vi "SVT Fractional Octave Filtering (N Ch).vi"(6 "reset filter (F)":bool, 7 "coerce to nearest standard midband frequency?":bool, 8 "error in (no error)":errorcluster, 9 "midband frequency":dbl, 10 "bandwidth":T1(ring), 11 "scaled signal(s)":waveform(dbl)[](array[waveform])) -> (0 "error out":errorcluster, 2 "actual midband frequency [Hz]":dbl, 3 "filtered signl(s)":waveform(dbl)[](array[waveform]), 4 "settled?":bool)   [LabVIEW 2017, in "SoundVib_Octave_2014 standard.lvlib"]
doc: "Performs fractional octave filtering on <B>scaled signal [EU]</B> in accordance with either the ANSI S1.11-2014 standard or the IEC 61260-1:2014 standard.\n\n \n\nYou can use this polymorphic VI to perform fractional octave filtering on a single channel or on N channels. The data type you wire to the <B>scaled signal [EU]</B> input determines the polymorphic instance to use."
uses:
  <vilib>/addons/Sound and Vibration/svt_Octave/SoundVib_Octave_2014 standard.lvlib
  <vilib>/addons/_NISVFA/_Shared subVIs/Controls/svc_Octave Standard.ctl
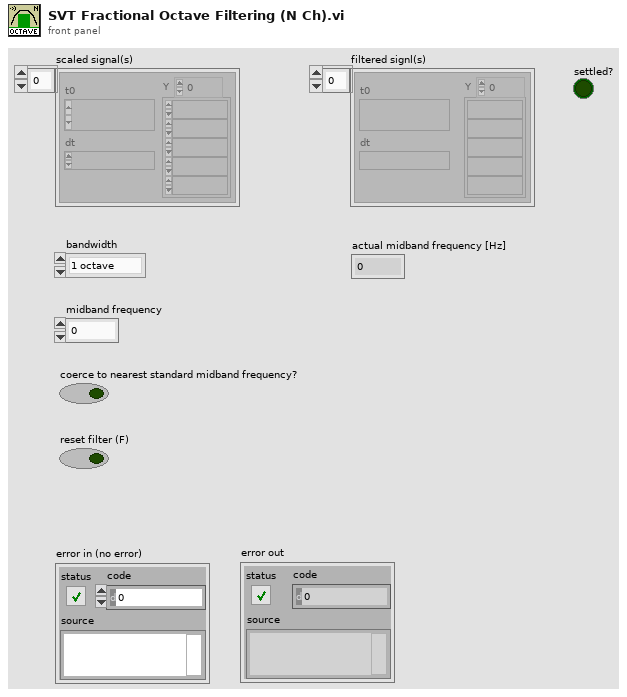
[diagram p1: front panel]
types:
  T1 = enum16{"1 octave", "1/3 octave", "1/6 octave", "1/12 octave", "1/24 octave"}
  T2 = typedef "svc_Octave Standard.ctl" = enum16{"ANSI S1.11", "IEC 61260"}
  T3 = cluster{"standard":T2, "bandwidth":enum16{"1 octave", "1/3 octave", "1/6 octave", "1/12 octave", "1/24 octave"}}
  T4 = cluster{"midband frequency":dbl, "coerce to nearest standard midband frequency?":bool}
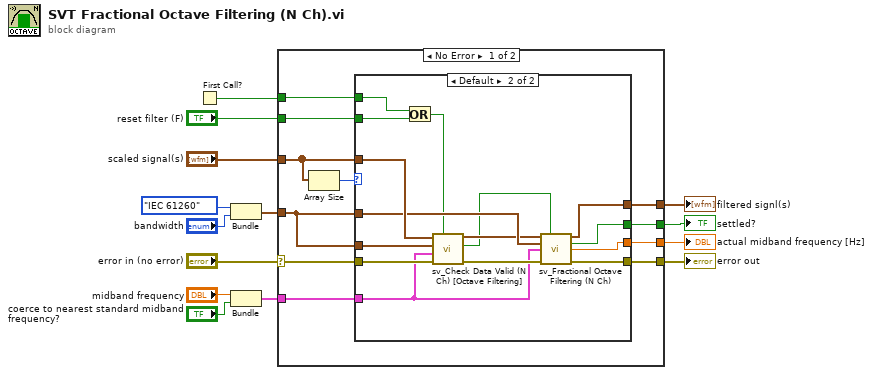
[diagram p0: block diagram]
diagram:
  n1 = First Call?() -> (First Call?: T/F=w11:bool)
  n2 = Bundle("standard"=svc_Octave_Standard."IEC 61260", "bandwidth"="bandwidth") -> (w5:T3)  [unwired: 1 in]
  n3 = Bundle("midband frequency"="midband frequency", "coerce to nearest standard midband frequency?"="coerce to nearest standard midband frequency?") -> (w2:T4)  [unwired: 1 in]
  n4 = case shown="No Error" "error in (no error)" {
    selector: "error in (no error)" -> [w25 w42]
    tunnel: [w16 w42] -> w13
    tunnel: "scaled signal(s)" -> [w24 _]
    tunnel: "reset filter (F)" -> [w22 _]
    tunnel: w5 -> [w20 _]
    tunnel: w2 -> [w19 _]
    tunnel: w11 -> [w21 _]
    tunnel: [w18 _] -> w8
    tunnel: [w17 _] -> w9
    tunnel: [w15 _] -> w1
    frame No Error {
      n5 = Array Size(array=w24) -> (size(s)=w23:i32)
      n6 = case shown="Default" w23 {
        tunnel: w25 -> [w26 w41]
        tunnel: w24 -> [_ w40]
        tunnel: w22 -> [_ w31]
        tunnel: w21 -> [_ w30]
        tunnel: w20 -> [_ w39]
        tunnel: w20 -> [_ w37]
        tunnel: w19 -> [_ w28]
        tunnel: [_ w34] -> w18
        tunnel: [_ w33] -> w17
        tunnel: [w26 w32] -> w16
        tunnel: [_ w27] -> w15
        frame 0 {
        }
        frame Default {
          n7 = Or(x=w30, y=w31) -> (x .or. y?=w29:bool)
          n8 = call <vilib>:"sv_Check Data Valid (N Ch) [Octave Filtering].vi"("reset filter (F)"=w29, "error in (no error)"=w41, "midband frequency setting"=w28, "1/n octave settings"=w39, "scaled signal(s)"=w40) -> ("error out"=w38:errorcluster, "reset filter"=w35:bool, "dup scaled signal(s)"=w36:waveform(dbl)[])  [unwired: 4 in]
          n9 = call <vilib>:"sv_Fractional Octave Filtering (N Ch).vi"("scaled signal(s) [EU]"=w36, "reset filter (F)"=w35, "1/n octave settings"=w37, "midband frequency setting"=w28, "error in (no error)"=w38) -> ("filtered signal(s) [EU]"=w34:waveform(dbl)[], "settled?"=w33:bool, "actual midband frequency [Hz]"=w27:dbl, "error out"=w32:errorcluster)  [unwired: 7 in]
        }
      }
    }
    frame Error {
    }
  }
  "error out" <- w13
  "settled?" <- w9
  "filtered signl(s)" <- w8
  "actual midband frequency [Hz]" <- w1
